vi "rs3 init spatial filter.vi"(8 "error in (no error)":errorcluster) -> (0 "error out":errorcluster, 1 "error spatial filter queue":u64, 2 "error spatial filter block":u64, 3 "error start processing":u64, 4 "spatial filter block":u64, 5 "spatial filter queue":u64)   [LabVIEW 2017, in "libRealSense3.lvlib"]
doc: "Initalizes the processing block and queue for the edge-preserving filter post-processing."
uses:
  libRealSense3.lvlib
panel:
  # "RS3 Init Spatial Filter"
  # "(C) Intel Corp.,  AGJ"
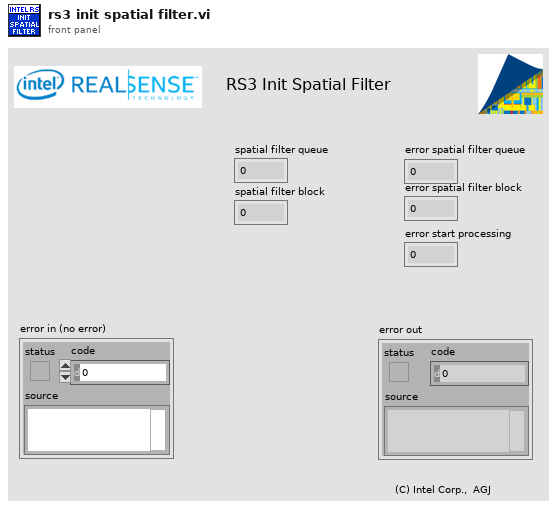
[diagram p1: front panel]
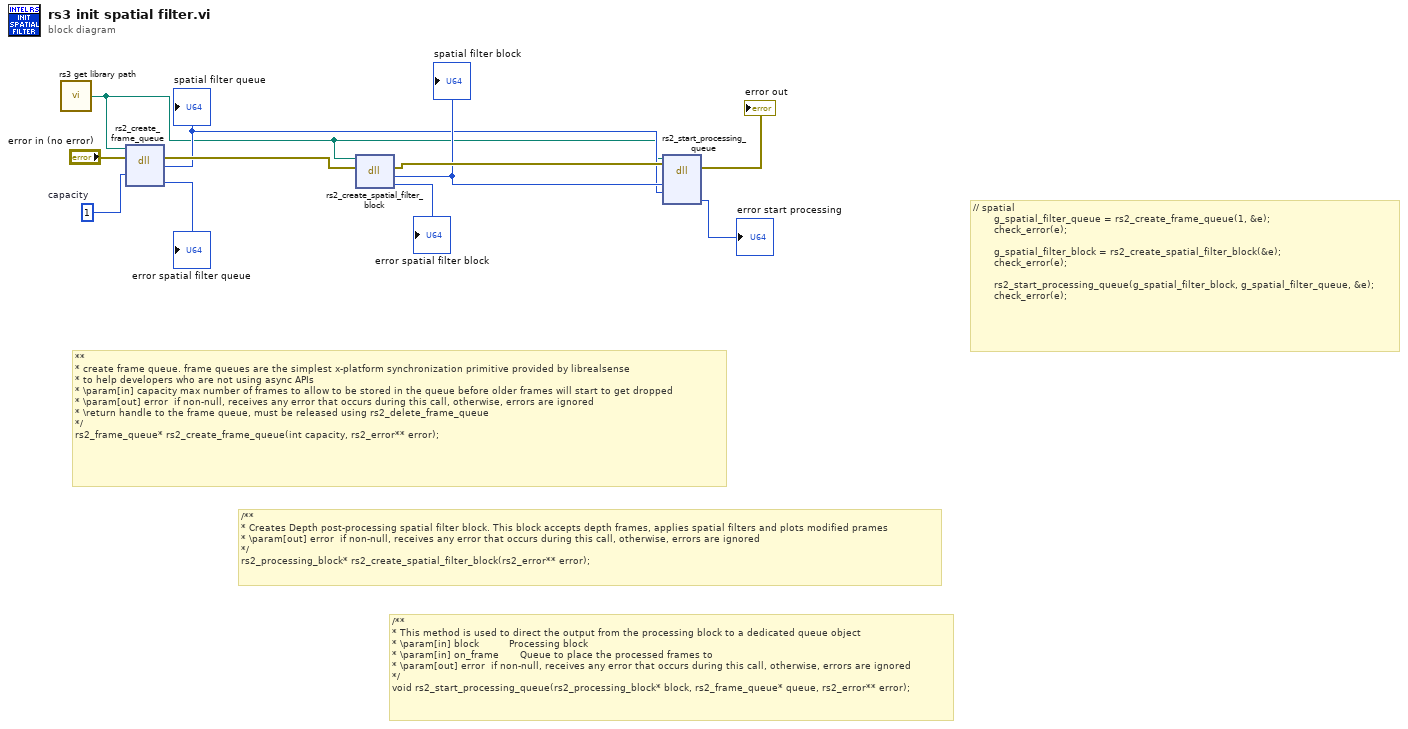
[diagram p0: block diagram]
diagram:
  w10 = 1  # capacity
  # "/**\n* Creates Depth post-processing spatial filter block. This block accepts depth frames, applies spatial filters and plots modified prames\n* \\param[out] error  if non-null, receives any error that occurs during this call, otherwise, errors are ignored\n*/\nrs2_processing_block* rs2_create_spatial_filter_block(rs2_error** error);"
  # "// spatial\n       g_spatial_filter_queue = rs2_create_frame_queue(1, &e);\n       check_error(e);\n\n       g_spatial_filter_block = rs2_create_spatial_filter_block(&e);\n       check_error(e);\n\n       rs2_start_processing_queue(g_spatial_filter_block, g_spatial_filter_queue, &e);\n       check_error(e);"
  # "/**\n* This method is used to direct the output from the processing block to a dedicated queue object\n* \\param[in] block          Processing block\n* \\param[in] on_frame       Queue to place the processed frames to\n* \\param[out] error  if non-null, receives any error that occurs during this call, otherwise, errors are ignored\n*/\nvoid rs2_start_processing_queue(rs2_processing_block* block, rs2_frame_queue* queue, rs2_error** error);"
  # "**\n* create frame queue. frame queues are the simplest x-platform synchronization primitive provided by librealsense\n* to help developers who are not using async APIs\n* \\param[in] capacity max number of frames to allow to be stored in the queue before older frames will start to get dropped\n* \\param[out] error  if non-null, receives any error that occurs during this call, otherwise, errors are ignored\n* \\return handle to the frame queue, must be released using rs2_delete_frame_queue\n*/\nrs2_frame_queue* rs2_create_frame_queue(int capacity, rs2_error** error);"
  n1 = call "rs3 get library path.vi"() -> ("Realsense 2 Library Path"=w1:path)
  n2 = dll-call lib="C:/Users/agrunnet/Documents/libRealSense6/realsense2.dll" fn="rs2_create_frame_queue"(path in=w1, error in="error in (no error)", "capacity"=w10) -> (error out=w8:errorcluster, "decimation filter queue"=w3:u64, "error"=→"error spatial filter queue":u64)  [unwired: 3 in, 1 out]
  "spatial filter queue" <- w3
  n3 = dll-call lib="C:/Users/agrunnet/Documents/libRealSense6/realsense2.dll" fn="rs2_create_spatial_filter_block"(path in=w1, error in=w8) -> (error out=w6:errorcluster, "spatial filter block"=w4:u64, "error"=→"error spatial filter block":u64)  [unwired: 2 in, 1 out]
  "spatial filter block" <- w4
  n4 = dll-call lib="C:/Users/agrunnet/Documents/libRealSense6/realsense2.dll" fn="rs2_start_processing_queue"(path in=w1, error in=w6, "processing block"=w4, "frame queue"=w3) -> (error out=→"error out":errorcluster, "error"=→"error start processing":u64)  [unwired: 5 in, 1 out]
